vi "nanocal -- nuclear schottky fit V7.vi"() -> ()   [LabVIEW 2021] (continued)
\"στN\" -> 0.000000000000    |>   , \n\"IDS0368_210908_RAW_cal__sam_\" ->   <|    \"ζ\" -> 0.021420270760   ,  \"τ1\" -> 0.018208454683   ,  \"τS\" -> 0.024985612374   ,  \"τN\" -> 0.002144760910   ,  \"τC\" -> 0.004931614434   ,  \"κ0\" -> 0.000000004254   ,  \"mm1\" -> 0.000086915042   ,  \"mm2\" -> 0.015826314138   ,  \"mm3\" -> 0.034938353162   ,  \"T\" -> 0.630000000000   ,  \"B\" -> 12.000000000000   ,  \"θ\" -> 60.000000000000   ,  \"Reoff\" -> -1204819.277108438310   ,  \"Imoff\" -> 0.000000000000   ,  \"στ1\" -> 0.000000000000   ,  \"στS\" -> 0.000000000000   ,  \"στN\" -> 0.000000000000    |>   , \n\"IDS0369_210908_RAW_cal__ref_\" ->   <|    \"ζ\" -> 0.022212344829   ,  \"τ1\" -> 0.017343641344   ,  \"τS\" -> 0.018001662092   ,  \"τN\" -> 0.000711569404   ,  \"τC\" -> 0.004309595418   ,  \"κ0\" -> 0.000000005439   ,  \"mm1\" -> 0.000076128819   ,  \"mm2\" -> 0.015699102017   ,  \"mm3\" -> 0.025006902173   ,  \"T\" -> 0.830000000000   ,  \"B\" -> 12.000000000000   ,  \"θ\" -> 60.000000000000   ,  \"Reoff\" -> 0.000000000000   ,  \"Imoff\" -> 0.000000000000   ,  \"στ1\" -> 0.000000000000   ,  \"στS\" -> 0.000000000000   ,  \"στN\" -> 0.000000000000    |>   , \n\"IDS0369_210908_RAW_cal__sam_\" ->   <|    \"ζ\" -> 0.014606512986   ,  \"τ1\" -> 0.019756664879   ,  \"τS\" -> 0.022303249954   ,  \"τN\" -> 0.001023812506   ,  \"τC\" -> 0.005490022400   ,  \"κ0\" -> 0.000000005866   ,  \"mm1\" -> 0.000063747249   ,  \"mm2\" -> 0.017921258799   ,  \"mm3\" -> 0.030929470731   ,  \"T\" -> 0.830000000000   ,  \"B\" -> 12.000000000000   ,  \"θ\" -> 60.000000000000   ,  \"Reoff\" -> -481927.710843376814   ,  \"Imoff\" -> 0.000000000000   ,  \"στ1\" -> 0.000000000000   ,  \"στS\" -> 0.000000000000   ,  \"στN\" -> 0.000000000000    |>   , \n\"IDS0370_210908_RAW_cal__ref_\" ->   <|    \"ζ\" -> 0.021569402950   ,  \"τ1\" -> 0.017921737944   ,  \"τS\" -> 0.015463128015   ,  \"τN\" -> 0.000390873619   ,  \"τC\" -> 0.004954240411   ,  \"κ0\" -> 0.000000007586   ,  \"mm1\" -> 0.000079935600   ,  \"mm2\" -> 0.016393641357   ,  \"mm3\" -> 0.022598364382   ,  \"T\" -> 1.130000000000   ,  \"B\" -> 12.000000000000   ,  \"θ\" -> 60.000000000000   ,  \"Reoff\" -> 0.000000000000   ,  \"Imoff\" -> 0.000000000000   ,  \"στ1\" -> 0.000000000000   ,  \"στS\" -> 0.000000000000   ,  \"στN\" -> 0.000000000000    |>   , \n\"IDS0370_210908_RAW_cal__sam_\" ->   <|    \"ζ\" -> 0.013427569249   ,  \"τ1\" -> 0.019934074843   ,  \"τS\" -> 0.019524726442   ,  \"τN\" -> 0.000513623253   ,  \"τC\" -> 0.005657316251   ,  \"κ0\" -> 0.000000008143   ,  \"mm1\" -> 0.000058424467   ,  \"mm2\" -> 0.018528796956   ,  \"mm3\" -> 0.027311585694   ,  \"T\" -> 1.130000000000   ,  \"B\" -> 12.000000000000   ,  \"θ\" -> 60.000000000000   ,  \"Reoff\" -> -481927.710843376814   ,  \"Imoff\" -> 0.000000000000   ,  \"στ1\" -> 0.000000000000   ,  \"στS\" -> 0.000000000000   ,  \"στN\" -> 0.000000000000    |>   , \n\"IDS0371_210908_RAW_cal__ref_\" ->   <|    \"ζ\" -> 0.020664849580   ,  \"τ1\" -> 0.018108723176   ,  \"τS\" -> 0.010299896170   ,  \"τN\" -> 0.000079818017   ,  \"τC\" -> 0.006259144045   ,  \"κ0\" -> 0.000000013130   ,  \"mm1\" -> 0.000079811267   ,  \"mm2\" -> 0.016056535433   ,  \"mm3\" -> 0.018825729941   ,  \"T\" -> 1.900000000000   ,  \"B\" -> 12.000000000000   ,  \"θ\" -> 60.000000000000   ,  \"Reoff\" -> 0.000000000000   ,  \"Imoff\" -> 0.000000000000   ,  \"στ1\" -> 0.000000000000   ,  \"στS\" -> 0.000000000000   ,  \"στN\" -> 0.000000000000    |>   , \n\"IDS0371_210908_RAW_cal__sam_\" ->   <|    \"ζ\" -> 0.009645933094   ,  \"τ1\" -> 0.020976887035   ,  \"τS\" -> 0.013140254521   ,  \"τN\" -> 0.000215522697   ,  \"τC\" -> 0.007317042194   ,  \"κ0\" -> 0.000000013897   ,  \"mm1\" -> 0.000045154509   ,  \"mm2\" -> 0.018728618799   ,  \"mm3\" -> 0.023004762073   ,  \"T\" -> 1.900000000000   ,  \"B\" -> 12.000000000000   ,  \"θ\" -> 60.000000000000   ,  \"Reoff\" -> -120481.927710846066   ,  \"Imoff\" -> 0.000000000000   ,  \"στ1\" -> 0.000000000000   ,  \"στS\" -> 0.000000000000   ,  \"στN\" -> 0.000000000000    |>   , \n\"IDS0372_210908_RAW_cal__ref_\" ->   <|    \"ζ\" -> 0.021592146431   ,  \"τ1\" -> 0.018093446545   ,  \"τS\" -> 0.007071841556   ,  \"τN\" -> 0.000029085223   ,  \"τC\" -> 0.005341206531   ,  \"κ0\" -> 0.000000023517   ,  \"mm1\" -> 0.000065243548   ,  \"mm2\" -> 0.012435446609   ,  \"mm3\" -> 0.018188213949   ,  \"T\" -> 3.110000000000   ,  \"B\" -> 12.000000000000   ,  \"θ\" -> 60.000000000000   ,  \"Reoff\" -> 0.000000000000   ,  \"Imoff\" -> 0.000000000000   ,  \"στ1\" -> 0.000000000000   ,  \"στS\" -> 0.000000000000   ,  \"στN\" -> 0.000000000000    |>   , \n\"IDS0372_210908_RAW_cal__sam_\" ->   <|    \"ζ\" -> 0.010006554735   ,  \"τ1\" -> 0.021193289022   ,  \"τS\" -> 0.010059776467   ,  \"τN\" -> 0.000092737128   ,  \"τC\" -> 0.005619947239   ,  \"κ0\" -> 0.000000024358   ,  \"mm1\" -> 0.000035931477   ,  \"mm2\" -> 0.015490366222   ,  \"mm3\" -> 0.021541043840   ,  \"T\" -> 3.110000000000   ,  \"B\" -> 12.000000000000   ,  \"θ\" -> 60.000000000000   ,  \"Reoff\" -> -120481.927710846066   ,  \"Imoff\" -> 0.000000000000   ,  \"στ1\" -> 0.000000000000   ,  \"στS\" -> 0.000000000000   ,  \"στN\" -> 0.000000000000    |>   , \n\"IDS0373_210908_RAW_cal__ref_\" ->   <|    \"ζ\" -> 0.028148688120   ,  \"τ1\" -> 0.012706961955   ,  \"τS\" -> 0.003881518121   ,  \"τN\" -> 0.000007160132   ,  \"τC\" -> 0.004346615253   ,  \"κ0\" -> 0.000000058313   ,  \"mm1\" -> 0.000057355729   ,  \"mm2\" -> 0.008266435527   ,  \"mm3\" -> 0.012727925396   ,  \"T\" -> 5.750000000000   ,  \"B\" -> 12.000000000000   ,  \"θ\" -> 60.000000000000   ,  \"Reoff\" -> 0.000000000000   ,  \"Imoff\" -> 0.000000000000   ,  \"στ1\" -> 0.000000000000   ,  \"στS\" -> 0.000000000000   ,  \"στN\" -> 0.000000000000    |>   , \n\"IDS0373_210908_RAW_cal__sam_\" ->   <|    \"ζ\" -> 0.009383547393   ,  \"τ1\" -> 0.021616814113   ,  \"τS\" -> 0.006389723126   ,  \"τN\" -> 0.000031102862   ,  \"τC\" -> 0.004593168461   ,  \"κ0\" -> 0.000000059183   ,  \"mm1\" -> 0.000024995592   ,  \"mm2\" -> 0.010985466166   ,  \"mm3\" -> 0.021680596929   ,  \"T\" -> 5.750000000000   ,  \"B\" -> 12.000000000000   ,  \"θ\" -> 60.000000000000   ,  \"Reoff\" -> -40000.000000000000   ,  \"Imoff\" -> 0.000000000000   ,  \"στ1\" -> 0.000000000000   ,  \"στS\" -> 0.000000000000   ,  \"στN\" -> 0.000000000000    |>   , \n\"IDS0377_210909_RAW_cal__ref_\" ->   <|    \"ζ\" -> 0.218126190413   ,  \"τ1\" -> 0.079838021846   ,  \"τS\" -> 0.035132352739   ,  \"τN\" -> 0.027061454869   ,  \"τC\" -> 0.001090107541   ,  \"κ0\" -> 0.000000001041   ,  \"mm1\" -> 0.000191179094   ,  \"mm2\" -> 0.026924011586   ,  \"mm3\" -> 0.129572844636   ,  \"T\" -> 0.197000000000   ,  \"B\" -> 8.000000000000   ,  \"θ\" -> 0.000000000000   ,  \"Reoff\" -> -30325301.204819276900   ,  \"Imoff\" -> 0.000000000000   ,  \"στ1\" -> 0.015121325479   ,  \"στS\" -> 0.001580446534   ,  \"στN\" -> 0.000000000000    |>   , \n\"IDS0377_210909_RAW_cal__sam_\" ->   <|    \"ζ\" -> 0.135798490691   ,  \"τ1\" -> 0.079257563336   ,  \"τS\" -> 0.046440970443   ,  \"τN\" -> 0.031537801980   ,  \"τC\" -> 0.001434159670   ,  \"κ0\" -> 0.000000001166   ,  \"mm1\" -> 0.000167444282   ,  \"mm2\" -> 0.031002991367   ,  \"mm3\" -> 0.138089459380   ,  \"T\" -> 0.197000000000   ,  \"B\" -> 8.000000000000   ,  \"θ\" -> 0.000000000000   ,  \"Reoff\" -> -18665662.650602411500   ,  \"Imoff\" -> 0.000000000000   ,  \"στ1\" -> 0.000000000000   ,  \"στS\" -> 0.000000000000   ,  \"στN\" -> 0.000000000000    |>   , \n\"IDS0378_210909_RAW_cal__ref_\" ->   <|    \"ζ\" -> 0.444552800957   ,  \"τ1\" -> 0.128860115614   ,  \"τS\" -> 0.109021040284   ,  \"τN\" -> 0.152308696924   ,  \"τC\" -> 0.001224528567   ,  \"κ0\" -> 0.000000000394   ,  \"mm1\" -> 0.000374811046   ,  \"mm2\" -> 0.044053094938   ,  \"mm3\" -> 0.463161342054   ,  \"T\" -> 0.122000000000   ,  \"B\" -> 8.000000000000   ,  \"θ\" -> 0.000000000000   ,  \"Reoff\" -> -133680722.891566262000   ,  \"Imoff\" -> 0.000000000000   ,  \"στ1\" -> 0.037474122176   ,  \"στS\" -> 0.013209355673   ,  \"στN\" -> 0.000000000000    |>   , \n\"IDS0378_210909_RAW_cal__sam_\" ->   <|    \"ζ\" -> 0.261650469875   ,  \"τ1\" -> 0.181870145043   ,  \"τS\" -> 0.168113301561   ,  \"τN\" -> 0.186965229666   ,  \"τC\" -> 0.001543998203   ,  \"κ0\" -> 0.000000000530   ,  \"mm1\" -> 0.000318362571   ,  \"mm2\" -> 0.069029342513   ,  \"mm3\" -> 0.562051433928   ,  \"T\" -> 0.122000000000   ,  \"B\" -> 8.000000000000   ,  \"θ\" -> 0.000000000000   ,  \"Reoff\" -> -63674698.795180723100   ,  \"Imoff\" -> 0.000000000000   ,  \"στ1\" -> 0.000000000000   ,  \"στS\" -> 0.000000000000   ,  \"στN\" -> 0.000000000000    |>   , \n\"IDS0379_210909_RAW_cal__ref_\" ->   <|    \"ζ\" -> 0.358941818136   ,  \"τ1\" -> 0.106560472447   ,  \"τS\" -> 0.062750754933   ,  \"τN\" -> 0.083489698826   ,  \"τC\" -> 0.001109485369   ,  \"κ0\" -> 0.000000000627   ,  \"mm1\" -> 0.000290253427   ,  \"mm2\" -> 0.033675860334   ,  \"mm3\" -> 0.272436112171   ,  \"T\" -> 0.148000000000   ,  \"B\" -> 8.000000000000   ,  \"θ\" -> 0.000000000000   ,  \"Reoff\" -> -71123493.975903615400   ,  \"Imoff\" -> 0.000000000000   ,  \"στ1\" -> 0.022940419447   ,  \"στS\" -> 0.005727663556   ,  \"στN\" -> 0.000000000000    |>   , \n\"IDS0379_210909_RAW_cal__sam_\" ->   <|    \"ζ\" -> 0.225699737863   ,  \"τ1\" -> 0.105340283181   ,  \"τS\" -> 0.080581728797   ,  \"τN\" -> 0.103261234048   ,  \"τC\" -> 0.001367459466   ,  \"κ0\" -> 0.000000000745   ,  \"mm1\" -> 0.000248975261   ,  \"mm2\" -> 0.035515573270   ,  \"mm3\" -> 0.296279465482   ,  \"T\" -> 0.148000000000   ,  \"B\" -> 8.000000000000   ,  \"θ\" -> 0.000000000000   ,  \"Reoff\" -> -47870481.927710846100   ,  \"Imoff\" -> 0.000000000000   ,  \"στ1\" -> 0.000000000000   ,  \"στS\" -> 0.000000000000   ,  \"στN\" -> 0.000000000000    |>   , \n\"IDS0380_210909_RAW_cal__ref_\" ->   <|    \"ζ\" -> 0.288906167077   ,  \"τ1\" -> 0.085305830839   ,  \"τS\" -> 0.050470435451   ,  \"τN\" -> 0.055834761417   ,  \"τC\" -> 0.001016000241   ,  \"κ0\" -> 0.000000000740   ,  \"mm1\" -> 0.000224990907   ,  \"mm2\" -> 0.028925222390   ,  \"mm3\" -> 0.194189041618   ,  \"T\" -> 0.168000000000   ,  \"B\" -> 8.000000000000   ,  \"θ\" -> 0.000000000000   ,  \"Reoff\" -> -51177710.843373492400   ,  \"Imoff\" -> 0.000000000000   ,  \"στ1\" -> 0.012964547595   ,  \"στS\" -> 0.003391652117   ,  \"στN\" -> 0.000000000000    |>   , \n\"IDS0380_210909_RAW_cal__sam_\" ->   <|    \"ζ\" -> 0.175751625392   ,  \"τ1\" -> 0.093635045165   ,  \"τS\" -> 0.061160146348   ,  \"τN\" -> 0.068664853746   ,  \"τC\" -> 0.001317909381   ,  \"κ0\" -> 0.000000000855   ,  \"mm1\" -> 0.000193962663   ,  \"mm2\" -> 0.031705338902   ,  \"mm3\" -> 0.215695607858   ,  \"T\" -> 0.168000000000   ,  \"B\" -> 8.000000000000   ,  \"θ\" -> 0.000000000000   ,  \"Reoff\" -> -37527108.433734938500   ,  \"Imoff\" -> 0.000000000000   ,  \"στ1\" -> 0.000000000000   ,  \"στS\" -> 0.000000000000   ,  \"στN\" -> 0.000000000000    |>   , \n\"IDS0381_210909_RAW_cal__ref_\" ->   <|    \"ζ\" -> 0.126929215903   ,  \"τ1\" -> 0.058068597672   ,  \"τS\" -> 0.026924833357   ,  \"τN\" -> 0.010980626621   ,  \"τC\" -> 0.001220007823   ,  \"κ0\" -> 0.000000001350   ,  \"mm1\" -> 0.000132654651   ,  \"mm2\" -> 0.023198783099   ,  \"mm3\" -> 0.078673938037   ,  \"T\" -> 0.250000000000   ,  \"B\" -> 8.000000000000   ,  \"θ\" -> 0.000000000000   ,  \"Reoff\" -> -15819277.108433738400   ,  \"Imoff\" -> 0.000000000000   ,  \"στ1\" -> 0.015255137459   ,  \"στS\" -> 0.000926224863   ,  \"στN\" -> 0.000000000000    |>   , \n\"IDS0381_210909_RAW_cal__sam_\" ->   <|    \"ζ\" -> 0.077362618852   ,  \"τ1\" -> 0.058638638627   ,  \"τS\" -> 0.035602410157   ,  \"τN\" -> 0.012932252536   ,  \"τC\" -> 0.001722606032   ,  \"κ0\" -> 0.000000001497   ,  \"mm1\" -> 0.000118727642   ,  \"mm2\" -> 0.027585733079   ,  \"mm3\" -> 0.084946215242   ,  \"T\" -> 0.250000000000   ,  \"B\" -> 8.000000000000   ,  \"θ\" -> 0.000000000000   ,  \"Reoff\" -> -9843373.493975907570   ,  \"Imoff\" -> 0.000000000000   ,  \"στ1\" -> 0.000000000000   ,  \"στS\" -> 0.000000000000   ,  \"στN\" -> 0.000000000000    |>   , \n\"IDS0382_210909_RAW_cal__ref_\" ->   <|    \"ζ\" -> 0.087213265729   ,  \"τ1\" -> 0.047168857768   ,  \"τS\" -> 0.024342516225   ,  \"τN\" -> 0.005605032155   ,  \"τC\" -> 0.001527723897   ,  \"κ0\" -> 0.000000001731   ,  \"mm1\" -> 0.000116341877   ,  \"mm2\" -> 0.022377768321   ,  \"mm3\" -> 0.058761843342   ,  \"T\" -> 0.300000000000   ,  \"B\" -> 8.000000000000   ,  \"θ\" -> 0.000000000000   ,  \"Reoff\" -> -7659638.554216861730   ,  \"Imoff\" -> 0.000000000000   ,  \"στ1\" -> 0.020347835445   ,  \"στS\" -> 0.000812834930   ,  \"στN\" -> 0.000000000000    |>   , \n\"IDS0382_210909_RAW_cal__sam_\" ->   <|    \"ζ\" -> 0.054029770351   ,  \"τ1\" -> 0.051440847518   ,  \"τS\" -> 0.032079834642   ,  \"τN\" -> 0.007150632998   ,  \"τC\" -> 0.002202148776   ,  \"κ0\" -> 0.000000001884   ,  \"mm1\" -> 0.000106291219   ,  \"mm2\" -> 0.027352636275   ,  \"mm3\" -> 0.067534149597   ,  \"T\" -> 0.300000000000   ,  \"B\" -> 8.000000000000   ,  \"θ\" -> 0.000000000000   ,  \"Reoff\" -> 0.000000000000   ,  \"Imoff\" -> 0.000000000000   ,  \"στ1\" -> 0.000000000000   ,  \"στS\" -> 0.000000000000   ,  \"στN\" -> 0.000000000000    |>   , \n\"IDS0383_210910_RAW_cal__ref_\" ->   <|    \"ζ\" -> 0.061570309960   ,  \"τ1\" -> 0.048310722428   ,  \"τS\" -> 0.023792409980   ,  \"τN\" -> 0.003687374315   ,  \"τC\" -> 0.001764707006   ,  \"κ0\" -> 0.000000002103   ,  \"mm1\" -> 0.000096006795   ,  \"mm2\" -> 0.023284907275   ,  \"mm3\" -> 0.055866238496   ,  \"T\" -> 0.360000000000   ,  \"B\" -> 8.000000000000   ,  \"θ\" -> 0.000000000000   ,  \"Reoff\" -> -3448979.591836734680   ,  \"Imoff\" -> 0.000000000000   ,  \"στ1\" -> 0.005347956996   ,  \"στS\" -> 0.000064354371   ,  \"στN\" -> 0.000271676879    |>   , \n\"IDS0383_210910_RAW_cal__sam_\" ->   <|    \"ζ\" -> 0.038341835326   ,  \"τ1\" -> 0.050866858713   ,  \"τS\" -> 0.030652081909   ,  \"τN\" -> 0.004623805952   ,  \"τC\" -> 0.002823684758   ,  \"κ0\" -> 0.000000002289   ,  \"mm1\" -> 0.000096034779   ,  \"mm2\" -> 0.028459102290   ,  \"mm3\" -> 0.061763836547   ,  \"T\" -> 0.360000000000   ,  \"B\" -> 8.000000000000   ,  \"θ\" -> 0.000000000000   ,  \"Reoff\" -> 0.000000000000   ,  \"Imoff\" -> 0.000000000000   ,  \"στ1\" -> 0.000000000000   ,  \"στS\" -> 0.000000000000   ,  \"στN\" -> 0.000000000000    |>   , \n\"IDS0384_210910_RAW_cal__ref_\" ->   <|    \"ζ\" -> 0.047202777788   ,  \"τ1\" -> 0.057863954153   ,  \"τS\" -> 0.024260411824   ,  \"τN\" -> 0.002654470453   ,  \"τC\" -> 0.001761397108   ,  \"κ0\" -> 0.000000002620   ,  \"mm1\" -> 0.000074450881   ,  \"mm2\" -> 0.024981139493   ,  \"mm3\" -> 0.062755100371   ,  \"T\" -> 0.430000000000   ,  \"B\" -> 8.000000000000   ,  \"θ\" -> 0.000000000000   ,  \"Reoff\" -> -3244897.959183673380   ,  \"Imoff\" -> 0.000000000000   ,  \"στ1\" -> 0.002290219569   ,  \"στS\" -> 0.000142046978   ,  \"στN\" -> 0.000047451996    |>   , \n\"IDS0384_210910_RAW_cal__sam_\" ->   <|    \"ζ\" -> 0.029950572027   ,  \"τ1\" -> 0.044923259835   ,  \"τS\" -> 0.030416367718   ,  \"τN\" -> 0.002541256331   ,  \"τC\" -> 0.003331031560   ,  \"κ0\" -> 0.000000002858   ,  \"mm1\" -> 0.000087776347   ,  \"mm2\" -> 0.029544080465   ,  \"mm3\" -> 0.052567158325   ,  \"T\" -> 0.430000000000   ,  \"B\" -> 8.000000000000   ,  \"θ\" -> 0.000000000000   ,  \"Reoff\" -> 0.000000000000   ,  \"Imoff\" -> 0.000000000000   ,  \"στ1\" -> 0.000000000000   ,  \"στS\" -> 0.000000000000   ,  \"στN\" -> 0.000000000000    |>   , \n\"IDS0385_210910_RAW_cal__ref_\" ->   <|    \"ζ\" -> 0.035475807726   ,  \"τ1\" -> 0.065760313158   ,  \"τS\" -> 0.025267783397   ,  \"τN\" -> 0.001609393203   ,  \"τC\" -> 0.002044840275   ,  \"κ0\" -> 0.000000003270   ,  \"mm1\" -> 0.000065128755   ,  \"mm2\" -> 0.026984383918   ,  \"mm3\" -> 0.068586306909   ,  \"T\" -> 0.530000000000   ,  \"B\" -> 8.000000000000   ,  \"θ\" -> 0.000000000000   ,  \"Reoff\" -> -1979591.836734693500   ,  \"Imoff\" -> 0.000000000000   ,  \"στ1\" -> 0.001664351640   ,  \"στS\" -> 0.000128238795   ,  \"στN\" -> 0.000017678335    |>   , \n\"IDS0385_210910_RAW_cal__sam_\" ->   <|    \"ζ\" -> 0.024600756648   ,  \"τ1\" -> 0.043958236582   ,  \"τS\" -> 0.031312750224   ,  \"τN\" -> 0.001348105931   ,  \"τC\" -> 0.003635120795   ,  \"κ0\" -> 0.000000003548   ,  \"mm1\" -> 0.000078569164   ,  \"mm2\" -> 0.031960914170   ,  \"mm3\" -> 0.049018211972   ,  \"T\" -> 0.530000000000   ,  \"B\" -> 8.000000000000   ,  \"θ\" -> 0.000000000000   ,  \"Reoff\" -> 0.000000000000   ,  \"Imoff\" -> 0.000000000000   ,  \"στ1\" -> 0.000000000000   ,  \"στS\" -> 0.000000000000   ,  \"στN\" -> 0.000000000000    |>   , \n\"IDS0386_210910_RAW_cal__ref_\" ->   <|    \"ζ\" -> 0.027356022248   ,  \"τ1\" -> 0.074378310089   ,  \"τS\" -> 0.026934589252   ,  \"τN\" -> 0.001226970514   ,  \"τC\" -> 0.002640125038   ,  \"κ0\" -> 0.000000003880   ,  \"mm1\" -> 0.000064313303   ,  \"mm2\" -> 0.029422406274   ,  \"mm3\" -> 0.076463663571   ,  \"T\" -> 0.630000000000   ,  \"B\" -> 8.000000000000   ,  \"θ\" -> 0.000000000000   ,  \"Reoff\" -> -918367.346938774919   ,  \"Imoff\" -> 0.000000000000   ,  \"στ1\" -> 0.006379756107   ,  \"στS\" -> 0.000121793583   ,  \"στN\" -> 0.000037562843    |>   , \n\"IDS0386_210910_RAW_cal__sam_\" ->   <|    \"ζ\" -> 0.019494767421   ,  \"τ1\" -> 0.040349410363   ,  \"τS\" -> 0.033202805363   ,  \"τN\" -> 0.000770756985   ,  \"τC\" -> 0.004303152006   ,  \"κ0\" -> 0.000000004241   ,  \"mm1\" -> 0.000073144130   ,  \"mm2\" -> 0.033928832906   ,  \"mm3\" -> 0.045286454378   ,  \"T\" -> 0.630000000000   ,  \"B\" -> 8.000000000000   ,  \"θ\" -> 0.000000000000   ,  \"Reoff\" -> 0.000000000000   ,  \"Imoff\" -> 0.000000000000   ,  \"στ1\" -> 0.000000000000   ,  \"στS\" -> 0.000000000000   ,  \"στN\" -> 0.000000000000    |>   , \n\"IDS0387_210910_RAW_cal__ref_\" ->   <|    \"ζ\" -> 0.019264160163   ,  \"τ1\" -> 0.087527894663   ,  \"τS\" -> 0.031057035415   ,  \"τN\" -> 0.000427139586   ,  \"τC\" -> 0.003758266843   ,  \"κ0\" -> 0.000000005420   ,  \"mm1\" -> 0.000063607457   ,  \"mm2\" -> 0.035059135271   ,  \"mm3\" -> 0.088254109969   ,  \"T\" -> 0.830000000000   ,  \"B\" -> 8.000000000000   ,  \"θ\" -> 0.000000000000   ,  \"Reoff\" -> -265306.122448978945   ,  \"Imoff\" -> 0.000000000000   ,  \"στ1\" -> 0.002293859023   ,  \"στS\" -> 0.000111457645   ,  \"στN\" -> 0.000005341576    |>   , \n\"IDS0387_210910_RAW_cal__sam_\" ->   <|    \"ζ\" -> 0.013958531253   ,  \"τ1\" -> 0.040449551738   ,  \"τS\" -> 0.038075316972   ,  \"τN\" -> 0.000218997482   ,  \"τC\" -> 0.005348147372   ,  \"κ0\" -> 0.000000005866   ,  \"mm1\" -> 0.000064761782   ,  \"mm2\" -> 0.038768935960   ,  \"mm3\" -> 0.045792848207   ,  \"T\" -> 0.830000000000   ,  \"B\" -> 8.000000000000   ,  \"θ\" -> 0.000000000000   ,  \"Reoff\" -> 0.000000000000   ,  \"Imoff\" -> 0.000000000000   ,  \"στ1\" -> 0.000000000000   ,  \"στS\" -> 0.000000000000   ,  \"στN\" -> 0.000000000000    |>   , \n\"IDS0388_210910_RAW_cal__ref_\" ->   <|    \"ζ\" -> 0.016281760718   ,  \"τ1\" -> 0.090583957743   ,  \"τS\" -> 0.040861551341   ,  \"τN\" -> 0.000285855584   ,  \"τC\" -> 0.003366386849   ,  \"κ0\" -> 0.000000007540   ,  \"mm1\" -> 0.000049943920   ,  \"mm2\" -> 0.044562023222   ,  \"mm3\" -> 0.091155736609   ,  \"T\" -> 1.130000000000   ,  \"B\" -> 8.000000000000   ,  \"θ\" -> 0.000000000000   ,  \"Reoff\" -> -428571.428571428172   ,  \"Imoff\" -> 0.000000000000   ,  \"στ1\" -> 0.001979710526   ,  \"στS\" -> 0.000154101040   ,  \"στN\" -> 0.000003400989    |>   , \n\"IDS0388_210910_RAW_cal__sam_\" ->   <|    \"ζ\" -> 0.011551866824   ,  \"τ1\" -> 0.040411227639   ,  \"τS\" -> 0.048181354691   ,  \"τN\" -> 0.000103559724   ,  \"τC\" -> 0.006232382617   ,  \"κ0\" -> 0.000000008161   ,  \"mm1\" -> 0.000063176601   ,  \"mm2\" -> 0.040126882627   ,  \"mm3\" -> 0.055296246344   ,  \"T\" -> 1.130000000000   ,  \"B\" -> 8.000000000000   ,  \"θ\" -> 0.000000000000   ,  \"Reoff\" -> 0.000000000000   ,  \"Imoff\" -> 0.000000000000   ,  \"στ1\" -> 0.000000000000   ,  \"στS\" -> 0.000000000000   ,  \"στN\" -> 0.000000000000    |>   , \n\"IDS0389_210910_RAW_cal__ref_\" ->   <|    \"ζ\" -> 0.019465629154   ,  \"τ1\" -> 0.035571135590   ,  \"τS\" -> 0.015266533820   ,  \"τN\" -> 0.000260285661   ,  \"τC\" -> 0.004529981538   ,  \"κ0\" -> 0.000000010200   ,  \"mm1\" -> 0.000067219896   ,  \"mm2\" -> 0.019697516293   ,  \"mm3\" -> 0.036165439730   ,  \"T\" -> 1.520000000000   ,  \"B\" -> 8.000000000000   ,  \"θ\" -> 0.000000000000   ,  \"Reoff\" -> -551020.408163265324   ,  \"Imoff\" -> 0.000000000000   ,  \"στ1\" -> 0.011471207658   ,  \"στS\" -> 0.000401132713   ,  \"στN\" -> 0.000048991456    |>   , \n\"IDS0389_210910_RAW_cal__sam_\" ->   <|    \"ζ\" -> 0.011148198813   ,  \"τ1\" -> 0.038849151842   ,  \"τS\" -> 0.019213865355   ,  \"τN\" -> 0.000045035153   ,  \"τC\" -> 0.005536708133   ,  \"κ0\" -> 0.000000011229   ,  \"mm1\" -> 0.000047596165   ,  \"mm2\" -> 0.024836509281   ,  \"mm3\" -> 0.038975357089   ,  \"T\" -> 1.520000000000   ,  \"B\" -> 8.000000000000   ,  \"θ\" -> 0.000000000000   ,  \"Reoff\" -> 0.000000000000   ,  \"Imoff\" -> 0.000000000000   ,  \"στ1\" -> 0.000000000000   ,  \"στS\" -> 0.000000000000   ,  \"στN\" -> 0.000000000000    |>   , \n\"IDS0390_210910_RAW_cal__ref_\" ->   <|    \"ζ\" -> 0.016838578105   ,  \"τ1\" -> 0.032747492196   ,  \"τS\" -> 0.011207679404   ,  \"τN\" -> 0.000117854318   ,  \"τC\" -> 0.003479559601   ,  \"κ0\" -> 0.000000013000   ,  \"mm1\" -> 0.000044274477   ,  \"mm2\" -> 0.014733756508   ,  \"mm3\" -> 0.032965260417   ,  \"T\" -> 1.900000000000   ,  \"B\" -> 8.000000000000   ,  \"θ\" -> 0.000000000000   ,  \"Reoff\" -> -346938.775510204024   ,  \"Imoff\" -> 0.000000000000   ,  \"στ1\" -> 0.005723858997   ,  \"στS\" -> 0.000088565552   ,  \"στN\" -> 0.000007225901    |>   , \n\"IDS0390_210910_RAW_cal__sam_\" ->   <|    \"ζ\" -> 0.010826949430   ,  \"τ1\" -> 0.038768037521   ,  \"τS\" -> 0.012925317198   ,  \"τN\" -> 0.000029157336   ,  \"τC\" -> 0.005196063884   ,  \"κ0\" -> 0.000000013864   ,  \"mm1\" -> 0.000039906108   ,  \"mm2\" -> 0.018195372076   ,  \"mm3\" -> 0.038823555195   ,  \"T\" -> 1.900000000000   ,  \"B\" -> 8.000000000000   ,  \"θ\" -> 0.000000000000   ,  \"Reoff\" -> 0.000000000000   ,  \"Imoff\" -> 0.000000000000   ,  \"στ1\" -> 0.000000000000   ,  \"στS\" -> 0.000000000000   ,  \"στN\" -> 0.000000000000    |>   , \n\"IDS0391_210910_RAW_cal__ref_\" ->   <|    \"ζ\" -> 0.014193901830   ,  \"τ1\" -> 0.092879337404   ,  \"τS\" -> 0.043047307828   ,  \"τN\" -> 0.000265545099   ,  \"τC\" -> 0.003595748456   ,  \"κ0\" -> 0.000000008330   ,  \"mm1\" -> 0.000046539933   ,  \"mm2\" -> 0.046932456699   ,  \"mm3\" -> 0.093423720537   ,  \"T\" -> 1.250000000000   ,  \"B\" -> 8.000000000000   ,  \"θ\" -> 0.000000000000   ,  \"Reoff\" -> -224489.795918366871   ,  \"Imoff\" -> 0.000000000000   ,  \"στ1\" -> 0.004842916086   ,  \"στS\" -> 0.000245036767   ,  \"στN\" -> 0.000003156227    |>   , \n\"IDS0391_210910_RAW_cal__sam_\" ->   <|    \"ζ\" -> 0.010962610928   ,  \"τ1\" -> 0.040398807374   ,  \"τS\" -> 0.051328988590   ,  \"τN\" -> 0.000070281011   ,  \"τC\" -> 0.006422533164   ,  \"κ0\" -> 0.000000008958   ,  \"mm1\" -> 0.000062039854   ,  \"mm2\" -> 0.040240103995   ,  \"mm3\" -> 0.058481936484   ,  \"T\" -> 1.250000000000   ,  \"B\" -> 8.000000000000   ,  \"θ\" -> 0.000000000000   ,  \"Reoff\" -> 0.000000000000   ,  \"Imoff\" -> 0.000000000000   ,  \"στ1\" -> 0.000000000000   ,  \"στS\" -> 0.000000000000   ,  \"στN\" -> 0.000000000000    |>   , \n\"IDS0392_210910_RAW_cal__ref_\" ->   <|    \"ζ\" -> 0.015915665125   ,  \"τ1\" -> 0.061543395288   ,  \"τS\" -> 0.031670398058   ,  \"τN\" -> 0.000248131167   ,  \"τC\" -> 0.003886930831   ,  \"κ0\" -> 0.000000009270   ,  \"mm1\" -> 0.000054412441   ,  \"mm2\" -> 0.035659745539   ,  \"mm3\" -> 0.062142701987   ,  \"T\" -> 1.390000000000   ,  \"B\" -> 8.000000000000   ,  \"θ\" -> 0.000000000000   ,  \"Reoff\" -> -224489.795918366871   ,  \"Imoff\" -> 0.000000000000   ,  \"στ1\" -> 0.005114709163   ,  \"στS\" -> 0.000350050575   ,  \"στN\" -> 0.000004808789    |>   , \n\"IDS0392_210910_RAW_cal__sam_\" ->   <|    \"ζ\" -> 0.010962610928   ,  \"τ1\" -> 0.040398807374   ,  \"τS\" -> 0.051328988590   ,  \"τN\" -> 0.000070281011   ,  \"τC\" -> 0.006422533164   ,  \"κ0\" -> 0.000000008958   ,  \"mm1\" -> 0.000062039854   ,  \"mm2\" -> 0.040240103995   ,  \"mm3\" -> 0.058481936484   ,  \"T\" -> 1.390000000000   ,  \"B\" -> 8.000000000000   ,  \"θ\" -> 0.000000000000   ,  \"Reoff\" -> 0.000000000000   ,  \"Imoff\" -> 0.000000000000   ,  \"στ1\" -> 0.000000000000   ,  \"στS\" -> 0.000000000000   ,  \"στN\" -> 0.000000000000    |>   , \n\"IDS0393_210910_RAW_cal__ref_\" ->   <|    \"ζ\" -> 0.014955256266   ,  \"τ1\" -> 0.026332624911   ,  \"τS\" -> 0.008352670277   ,  \"τN\" -> 0.000164111809   ,  \"τC\" -> 0.002903513034   ,  \"κ0\" -> 0.000000023300   ,  \"mm1\" -> 0.000031957834   ,  \"mm2\" -> 0.011225492804   ,  \"mm3\" -> 0.026622840052   ,  \"T\" -> 3.110000000000   ,  \"B\" -> 8.000000000000   ,  \"θ\" -> 0.000000000000   ,  \"Reoff\" -> -183673.469387754798   ,  \"Imoff\" -> 0.000000000000   ,  \"στ1\" -> 0.001054663608   ,  \"στS\" -> 0.000052081378   ,  \"στN\" -> 0.000002015225    |>   , \n\"IDS0393_210910_RAW_cal__sam_\" ->   <|    \"ζ\" -> 0.010962610928   ,  \"τ1\" -> 0.040398807374   ,  \"τS\" -> 0.051328988590   ,  \"τN\" -> 0.000070281011   ,  \"τC\" -> 0.006422533164   ,  \"κ0\" -> 0.000000008958   ,  \"mm1\" -> 0.000062039854   ,  \"mm2\" -> 0.040240103995   ,  \"mm3\" -> 0.058481936484   ,  \"T\" -> 3.110000000000   ,  \"B\" -> 8.000000000000   ,  \"θ\" -> 0.000000000000   ,  \"Reoff\" -> 0.000000000000   ,  \"Imoff\" -> 0.000000000000   ,  \"στ1\" -> 0.000000000000   ,  \"στS\" -> 0.000000000000   ,  \"στN\" -> 0.000000000000    |>   , \n\"IDS0394_210910_RAW_cal__ref_\" ->   <|    \"ζ\" -> 0.016050939839   ,  \"τ1\" -> 0.020478636674   ,  \"τS\" -> 0.005312059468   ,  \"τN\" -> 0.000195533635   ,  \"τC\" -> 0.002460552068   ,  \"κ0\" -> 0.000000057800   ,  \"mm1\" -> 0.000026789678   ,  \"mm2\" -> 0.007711278862   ,  \"mm3\" -> 0.020797115351   ,  \"T\" -> 5.750000000000   ,  \"B\" -> 8.000000000000   ,  \"θ\" -> 0.000000000000   ,  \"Reoff\" -> -61224.489795917645   ,  \"Imoff\" -> 0.000000000000   ,  \"στ1\" -> 0.004716029121   ,  \"στS\" -> 0.000047047015   ,  \"στN\" -> 0.000018531547    |>   , \n\"IDS0394_210910_RAW_cal__sam_\" ->   <|    \"ζ\" -> 0.010962610928   ,  \"τ1\" -> 0.040398807374   ,  \"τS\" -> 0.051328988590   ,  \"τN\" -> 0.000070281011   ,  \"τC\" -> 0.006422533164   ,  \"κ0\" -> 0.000000008958   ,  \"mm1\" -> 0.000062039854   ,  \"mm2\" -> 0.040240103995   ,  \"mm3\" -> 0.058481936484   ,  \"T\" -> 5.750000000000   ,  \"B\" -> 8.000000000000   ,  \"θ\" -> 0.000000000000   ,  \"Reoff\" -> 0.000000000000   ,  \"Imoff\" -> 0.000000000000   ,  \"στ1\" -> 0.000000000000   ,  \"στS\" -> 0.000000000000   ,  \"στN\" -> 0.000000000000    |>   , \n\"IDS0395_210910_RAW_cal__ref_\" ->   <|    \"ζ\" -> 0.014321636830   ,  \"τ1\" -> 0.097433211743   ,  \"τS\" -> 0.042062236733   ,  \"τN\" -> 0.000244628908   ,  \"τC\" -> 0.003645191846   ,  \"κ0\" -> 0.000000008580   ,  \"mm1\" -> 0.000047465439   ,  \"mm2\" -> 0.046040095215   ,  \"mm3\" -> 0.097903612141   ,  \"T\" -> 1.310000000000   ,  \"B\" -> 8.000000000000   ,  \"θ\" -> 0.000000000000   ,  \"Reoff\" -> -224489.795918366871   ,  \"Imoff\" -> 0.000000000000   ,  \"στ1\" -> 0.012889257014   ,  \"στS\" -> 0.000375170132   ,  \"στN\" -> 0.000004995458    |>   , \n\"IDS0395_210910_RAW_cal__sam_\" ->   <|    \"ζ\" -> 0.010962610928   ,  \"τ1\" -> 0.040398807374   ,  \"τS\" -> 0.051328988590   ,  \"τN\" -> 0.000070281011   ,  \"τC\" -> 0.006422533164   ,  \"κ0\" -> 0.000000008958   ,  \"mm1\" -> 0.000062039854   ,  \"mm2\" -> 0.040240103995   ,  \"mm3\" -> 0.058481936484   ,  \"T\" -> 1.310000000000   ,  \"B\" -> 8.000000000000   ,  \"θ\" -> 0.000000000000   ,  \"Reoff\" -> 0.000000000000   ,  \"Imoff\" -> 0.000000000000   ,  \"στ1\" -> 0.000000000000   ,  \"στS\" -> 0.000000000000   ,  \"στN\" -> 0.000000000000    |>   , \n\"IDS0407_220525_RAW_cal__ref_\" ->   <|    \"ζ\" -> 0.185082039484   ,  \"τ1\" -> 0.020077955798   ,  \"τS\" -> 0.012960000170   ,  \"τN\" -> 0.004537831890   ,  \"τC\" -> 0.001384950660   ,  \"κ0\" -> 0.000000000762   ,  \"mm1\" -> 0.000200762639   ,  \"mm2\" -> 0.010571518349   ,  \"mm3\" -> 0.031426991974   ,  \"T\" -> 0.200000000000   ,  \"B\" -> 0.000000000000   ,  \"θ\" -> 0.000000000000   ,  \"Reoff\" -> -36285714.285714283600   ,  \"Imoff\" -> 0.000000000000   ,  \"στ1\" -> 0.006379909660   ,  \"στS\" -> 0.001208627120   ,  \"στN\" -> 0.001505491002    |>   , \n\"IDS0407_220525_RAW_cal__sam_\" ->   <|    \"ζ\" -> 0.107728168967   ,  \"τ1\" -> 0.019656327090   ,  \"τS\" -> 0.016556579862   ,  \"τN\" -> 0.004758156992   ,  \"τC\" -> 0.001123654800   ,  \"κ0\" -> 0.000000000861   ,  \"mm1\" -> 0.000103510666   ,  \"mm2\" -> 0.011667063931   ,  \"mm3\" -> 0.032620341720   ,  \"T\" -> 0.200000000000   ,  \"B\" -> 0.000000000000   ,  \"θ\" -> 0.000000000000   ,  \"Reoff\" -> -36285714.285714283600   ,  \"Imoff\" -> 0.000000000000   ,  \"στ1\" -> 0.009912643228   ,  \"στS\" -> 0.001520300197   ,  \"στN\" -> 0.002063455636    |>   , \n\"IDS0408_220525_RAW_cal__ref_\" ->   <|    \"ζ\" -> 0.136667515629   ,  \"τ1\" -> 0.013397105369   ,  \"τS\" -> 0.011359937502   ,  \"τN\" -> 0.003646822051   ,  \"τC\" -> 0.000857952267   ,  \"κ0\" -> 0.000000001040   ,  \"mm1\" -> 0.000097405399   ,  \"mm2\" -> 0.007836148791   ,  \"mm3\" -> 0.023379199545   ,  \"T\" -> 0.250000000000   ,  \"B\" -> 0.000000000000   ,  \"θ\" -> 0.000000000000   ,  \"Reoff\" -> -36285714.285714283600   ,  \"Imoff\" -> 0.000000000000   ,  \"στ1\" -> 0.003212907599   ,  \"στS\" -> 0.000580541661   ,  \"στN\" -> 0.000811635824    |>   , \n\"IDS0408_220525_RAW_cal__sam_\" ->   <|    \"ζ\" -> 0.086238207773   ,  \"τ1\" -> 0.018354133297   ,  \"τS\" -> 0.015001679768   ,  \"τN\" -> 0.004138272742   ,  \"τC\" -> 0.001377972360   ,  \"κ0\" -> 0.000000001190   ,  \"mm1\" -> 0.000101440698   ,  \"mm2\" -> 0.010941566515   ,  \"mm3\" -> 0.029479646155   ,  \"T\" -> 0.250000000000   ,  \"B\" -> 0.000000000000   ,  \"θ\" -> 0.000000000000   ,  \"Reoff\" -> -26000000.000000000000   ,  \"Imoff\" -> 0.000000000000   ,  \"στ1\" -> 0.004778614510   ,  \"στS\" -> 0.000718856892   ,  \"στN\" -> 0.001132000122    |>   , \n\"IDS0409_220525_RAW_cal__ref_\" ->   <|    \"ζ\" -> 0.104307058542   ,  \"τ1\" -> 0.013891003970   ,  \"τS\" -> 0.010729497189   ,  \"τN\" -> 0.003200228441   ,  \"τC\" -> 0.001175856975   ,  \"κ0\" -> 0.000000001350   ,  \"mm1\" -> 0.000101815669   ,  \"mm2\" -> 0.008053188158   ,  \"mm3\" -> 0.022294551454   ,  \"T\" -> 0.300000000000   ,  \"B\" -> 0.000000000000   ,  \"θ\" -> 0.000000000000   ,  \"Reoff\" -> -17138775.510204076800   ,  \"Imoff\" -> 0.000000000000   ,  \"στ1\" -> 0.002172719957   ,  \"στS\" -> 0.000093763545   ,  \"στN\" -> 0.000355038458    |>   , \n\"IDS0409_220525_RAW_cal__sam_\" ->   <|    \"ζ\" -> 0.056561047780   ,  \"τ1\" -> 0.014299678758   ,  \"τS\" -> 0.013769239985   ,  \"τN\" -> 0.003071380883   ,  \"τC\" -> 0.001651608796   ,  \"κ0\" -> 0.000000001520   ,  \"mm1\" -> 0.000079784788   ,  \"mm2\" -> 0.009566648569   ,  \"mm3\" -> 0.024097998227   ,  \"T\" -> 0.300000000000   ,  \"B\" -> 0.000000000000   ,  \"θ\" -> 0.000000000000   ,  \"Reoff\" -> -9836734.693877555430   ,  \"Imoff\" -> 0.000000000000   ,  \"στ1\" -> 0.019869000982   ,  \"στS\" -> 0.002333902836   ,  \"στN\" -> 0.003131938876    |>   , \n\"IDS0410_220525_RAW_cal__ref_\" ->   <|    \"ζ\" -> 0.219464822230   ,  \"τ1\" -> 0.031337357476   ,  \"τS\" -> 0.015000716363   ,  \"τN\" -> 0.006678392144   ,  \"τC\" -> 0.001899192874   ,  \"κ0\" -> 0.000000000590   ,  \"mm1\" -> 0.000314430704   ,  \"mm2\" -> 0.013625332075   ,  \"mm3\" -> 0.045733697773   ,  \"T\" -> 0.170000000000   ,  \"B\" -> 0.000000000000   ,  \"θ\" -> 0.000000000000   ,  \"Reoff\" -> -36285714.285714283600   ,  \"Imoff\" -> 0.000000000000   ,  \"στ1\" -> 0.008766031660   ,  \"στS\" -> 0.001214804635   ,  \"στN\" -> 0.000507557698    |>   , \n\"IDS0410_220525_RAW_cal__sam_\" ->   <|    \"ζ\" -> 0.124885425459   ,  \"τ1\" -> 0.026966294273   ,  \"τS\" -> 0.017799663974   ,  \"τN\" -> 0.005835531331   ,  \"τC\" -> 0.001338388753   ,  \"κ0\" -> 0.000000000710   ,  \"mm1\" -> 0.000140185240   ,  \"mm2\" -> 0.014066781222   ,  \"mm3\" -> 0.040684603290   ,  \"T\" -> 0.170000000000   ,  \"B\" -> 0.000000000000   ,  \"θ\" -> 0.000000000000   ,  \"Reoff\" -> -36285714.285714283600   ,  \"Imoff\" -> 0.000000000000   ,  \"στ1\" -> 0.125291630718   ,  \"στS\" -> 0.008513087182   ,  \"στN\" -> 0.016544280517    |>   , \n\"IDS0411_220525_RAW_cal__ref_\" ->   <|    \"ζ\" -> 0.246063307500   ,  \"τ1\" -> 0.040789582366   ,  \"τS\" -> 0.016746728194   ,  \"τN\" -> 0.008396680213   ,  \"τC\" -> 0.002075116481   ,  \"κ0\" -> 0.000000000510   ,  \"mm1\" -> 0.000378838091   ,  \"mm2\" -> 0.015895872639   ,  \"mm3\" -> 0.057920266758   ,  \"T\" -> 0.150000000000   ,  \"B\" -> 0.000000000000   ,  \"θ\" -> 0.000000000000   ,  \"Reoff\" -> -36285714.285714283600   ,  \"Imoff\" -> 0.000000000000   ,  \"στ1\" -> 0.014361572724   ,  \"στS\" -> 0.001491857642   ,  \"στN\" -> 0.002913772081    |>   , \n\"IDS0411_220525_RAW_cal__sam_\" ->   <|    \"ζ\" -> 0.135609092663   ,  \"τ1\" -> 0.033619209304   ,  \"τS\" -> 0.020242350677   ,  \"τN\" -> 0.009065316224   ,  \"τC\" -> 0.001338388753   ,  \"κ0\" -> 0.000000000610   ,  \"mm1\" -> 0.000151964902   ,  \"mm2\" -> 0.015437467353   ,  \"mm3\" -> 0.052650218819   ,  \"T\" -> 0.150000000000   ,  \"B\" -> 0.000000000000   ,  \"θ\" -> 0.000000000000   ,  \"Reoff\" -> -36285714.285714283600   ,  \"Imoff\" -> 0.000000000000   ,  \"στ1\" -> 0.012006153279   ,  \"στS\" -> 0.002506054906   ,  \"στN\" -> 0.002275285607    |>   , \n\"IDS0412_220525_RAW_cal__ref_\" ->   <|    \"ζ\" -> 0.277356261420   ,  \"τ1\" -> 0.054222210065   ,  \"τS\" -> 0.019549661431   ,  \"τN\" -> 0.015941590375   ,  \"τC\" -> 0.002328566298   ,  \"κ0\" -> 0.000000000395   ,  \"mm1\" -> 0.000470356932   ,  \"mm2\" -> 0.017304710415   ,  \"mm3\" -> 0.084110681736   ,  \"T\" -> 0.120000000000   ,  \"B\" -> 0.000000000000   ,  \"θ\" -> 0.000000000000   ,  \"Reoff\" -> -36285714.285714283600   ,  \"Imoff\" -> 0.000000000000   ,  \"στ1\" -> 0.003181743448   ,  \"στS\" -> 0.002733063927   ,  \"στN\" -> 0.005931070528    |>   , \n\"IDS0412_220525_RAW_cal__sam_\" ->   <|    \"ζ\" -> 0.141872667412   ,  \"τ1\" -> 0.045522682755   ,  \"τS\" -> 0.024683404671   ,  \"τN\" -> 0.014187266741   ,  \"τC\" -> 0.001029575567   ,  \"κ0\" -> 0.000000000485   ,  \"mm1\" -> 0.000123931838   ,  \"mm2\" -> 0.018251391889   ,  \"mm3\" -> 0.072562291843   ,  \"T\" -> 0.120000000000   ,  \"B\" -> 0.000000000000   ,  \"θ\" -> 0.000000000000   ,  \"Reoff\" -> -36285714.285714283600   ,  \"Imoff\" -> 0.000000000000   ,  \"στ1\" -> 0.019575103663   ,  \"στS\" -> 0.006297786999   ,  \"στN\" -> 0.007663344539    |>   , \n\"IDS0413_220525_RAW_cal__ref_\" ->   <|    \"ζ\" -> 0.078611813010   ,  \"τ1\" -> 0.009498211202   ,  \"τS\" -> 0.010412643153   ,  \"τN\" -> 0.002291796830   ,  \"τC\" -> 0.001202807939   ,  \"κ0\" -> 0.000000001750   ,  \"mm1\" -> 0.000079680552   ,  \"mm2\" -> 0.006634465733   ,  \"mm3\" -> 0.017690031900   ,  \"T\" -> 0.360000000000   ,  \"B\" -> 0.000000000000   ,  \"θ\" -> 0.000000000000   ,  \"Reoff\" -> -10542857.142857149200   ,  \"Imoff\" -> 0.000000000000   ,  \"στ1\" -> 0.000920556157   ,  \"στS\" -> 0.001775574992   ,  \"στN\" -> 0.000302317441    |>   , \n\"IDS0413_220525_RAW_cal__sam_\" ->   <|    \"ζ\" -> 0.044690907244   ,  \"τ1\" -> 0.013320614253   ,  \"τS\" -> 0.013760942515   ,  \"τN\" -> 0.002327045716   ,  \"τC\" -> 0.001523256988   ,  \"κ0\" -> 0.000000001960   ,  \"mm1\" -> 0.000059136229   ,  \"mm2\" -> 0.009591413737   ,  \"mm3\" -> 0.022000296296   ,  \"T\" -> 0.360000000000   ,  \"B\" -> 0.000000000000   ,  \"θ\" -> 0.000000000000   ,  \"Reoff\" -> -7142857.142857141800   ,  \"Imoff\" -> 0.000000000000   ,  \"στ1\" -> 0.002601583253   ,  \"στS\" -> 0.000378567326   ,  \"στN\" -> 0.000355149378    |>   , \n\"IDS0414_220525_RAW_cal__ref_\" ->   <|    \"ζ\" -> 0.062609276926   ,  \"τ1\" -> 0.008775091045   ,  \"τS\" -> 0.010532925062   ,  \"τN\" -> 0.001963246111   ,  \"τC\" -> 0.001185562237   ,  \"κ0\" -> 0.000000002220   ,  \"mm1\" -> 0.000063480840   ,  \"mm2\" -> 0.006468821738   ,  \"mm3\" -> 0.016706898118   ,  \"T\" -> 0.430000000000   ,  \"B\" -> 0.000000000000   ,  \"θ\" -> 0.000000000000   ,  \"Reoff\" -> -7657142.857142858210   ,  \"Imoff\" -> 0.000000000000   ,  \"στ1\" -> 0.001587412963   ,  \"στS\" -> 0.001748149515   ,  \"στN\" -> 0.000451539809    |>   , \n\"IDS0414_220525_RAW_cal__sam_\" ->   <|    \"ζ\" -> 0.036206503728   ,  \"τ1\" -> 0.010323598347   ,  \"τS\" -> 0.013793333734   ,  \"τN\" -> 0.001947462554   ,  \"τC\" -> 0.001576858934   ,  \"κ0\" -> 0.000000002450   ,  \"mm1\" -> 0.000049775806   ,  \"mm2\" -> 0.008169881573   ,  \"mm3\" -> 0.019991515390   ,  \"T\" -> 0.430000000000   ,  \"B\" -> 0.000000000000   ,  \"θ\" -> 0.000000000000   ,  \"Reoff\" -> -5183673.469387754800   ,  \"Imoff\" -> 0.000000000000   ,  \"στ1\" -> 0.000547128250   ,  \"στS\" -> 0.000218959699   ,  \"στN\" -> 0.000102085685    |>   , \n\"IDS0415_220525_RAW_cal__ref_\" ->   <|    \"ζ\" -> 0.048185231284   ,  \"τ1\" -> 0.008100929282   ,  \"τS\" -> 0.011138600782   ,  \"τN\" -> 0.001553114505   ,  \"τC\" -> 0.001221442635   ,  \"κ0\" -> 0.000000002870   ,  \"mm1\" -> 0.000051029801   ,  \"mm2\" -> 0.006456930010   ,  \"mm3\" -> 0.016117680629   ,  \"T\" -> 0.530000000000   ,  \"B\" -> 0.000000000000   ,  \"θ\" -> 0.000000000000   ,  \"Reoff\" -> -5600000.000000000000   ,  \"Imoff\" -> 0.000000000000   ,  \"στ1\" -> 0.001291082516   ,  \"στS\" -> 0.001596793517   ,  \"στN\" -> 0.000325645365    |>   , \n\"IDS0415_220525_RAW_cal__sam_\" ->   <|    \"ζ\" -> 0.029049723552   ,  \"τ1\" -> 0.007716049820   ,  \"τS\" -> 0.014447051972   ,  \"τN\" -> 0.001246053989   ,  \"τC\" -> 0.001554051920   ,  \"κ0\" -> 0.000000003200   ,  \"mm1\" -> 0.000039813384   ,  \"mm2\" -> 0.006805314073   ,  \"mm3\" -> 0.018573960634   ,  \"T\" -> 0.530000000000   ,  \"B\" -> 0.000000000000   ,  \"θ\" -> 0.000000000000   ,  \"Reoff\" -> -3959183.673469387000   ,  \"Imoff\" -> 0.000000000000   ,  \"στ1\" -> 0.000764801064   ,  \"στS\" -> 0.002293201092   ,  \"στN\" -> 0.000221114317    |>   , \n\"IDS0416_220525_RAW_cal__ref_\" ->   <|    \"ζ\" -> 0.039880135587   ,  \"τ1\" -> 0.006886163932   ,  \"τS\" -> 0.012166095681   ,  \"τN\" -> 0.001127457198   ,  \"τC\" -> 0.001222704242   ,  \"κ0\" -> 0.000000003530   ,  \"mm1\" -> 0.000042889516   ,  \"mm2\" -> 0.005990891230   ,  \"mm3\" -> 0.015898788997   ,  \"T\" -> 0.630000000000   ,  \"B\" -> 0.000000000000   ,  \"θ\" -> 0.000000000000   ,  \"Reoff\" -> -4057142.857142858210   ,  \"Imoff\" -> 0.000000000000   ,  \"στ1\" -> 0.001015861741   ,  \"στS\" -> 0.001565951598   ,  \"στN\" -> 0.000225145356    |>   , \n\"IDS0416_220525_RAW_cal__sam_\" ->   <|    \"ζ\" -> 0.022998692784   ,  \"τ1\" -> 0.007393021158   ,  \"τS\" -> 0.015620230500   ,  \"τN\" -> 0.001040733682   ,  \"τC\" -> 0.001765774011   ,  \"κ0\" -> 0.000000003911   ,  \"mm1\" -> 0.000035818495   ,  \"mm2\" -> 0.006739334009   ,  \"mm3\" -> 0.019427787243   ,  \"T\" -> 0.630000000000   ,  \"B\" -> 0.000000000000   ,  \"θ\" -> 0.000000000000   ,  \"Reoff\" -> -2408163.265306121670   ,  \"Imoff\" -> 0.000000000000   ,  \"στ1\" -> 0.000980763421   ,  \"στS\" -> 0.002016923628   ,  \"στN\" -> 0.000219391445    |>   , \n\"IDS0417_220525_RAW_cal__ref_\" ->   <|    \"ζ\" -> 0.032750219175   ,  \"τ1\" -> 0.005623693280   ,  \"τS\" -> 0.015325743160   ,  \"τN\" -> 0.000717738154   ,  \"τC\" -> 0.001196295790   ,  \"κ0\" -> 0.000000004900   ,  \"mm1\" -> 0.000035343333   ,  \"mm2\" -> 0.005288786846   ,  \"mm3\" -> 0.018064767734   ,  
